vi "Graph.vi"() -> ()   [LabVIEW 2018]
panel:
  in  "Tab Control":enum32{"Page 1", "Page 2"}(tab)
  out "XY Graph":cluster{"Array Ox":dbl[], "Array Oy":dbl[]}[](graph)
  in  "Button":bool
  out "Boolean":bool
  in  "Combo Box":string(combo)
  in  "Stop":bool
  in  "Start":bool
  in  "Config":bool
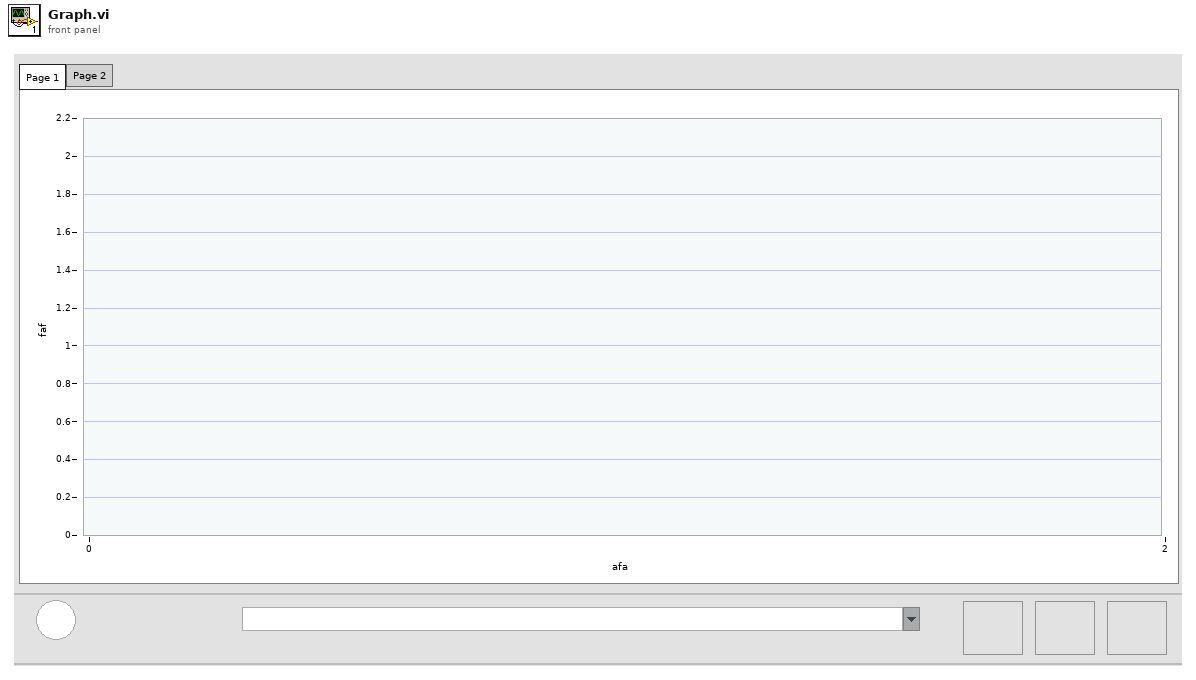
[diagram p1: front panel]
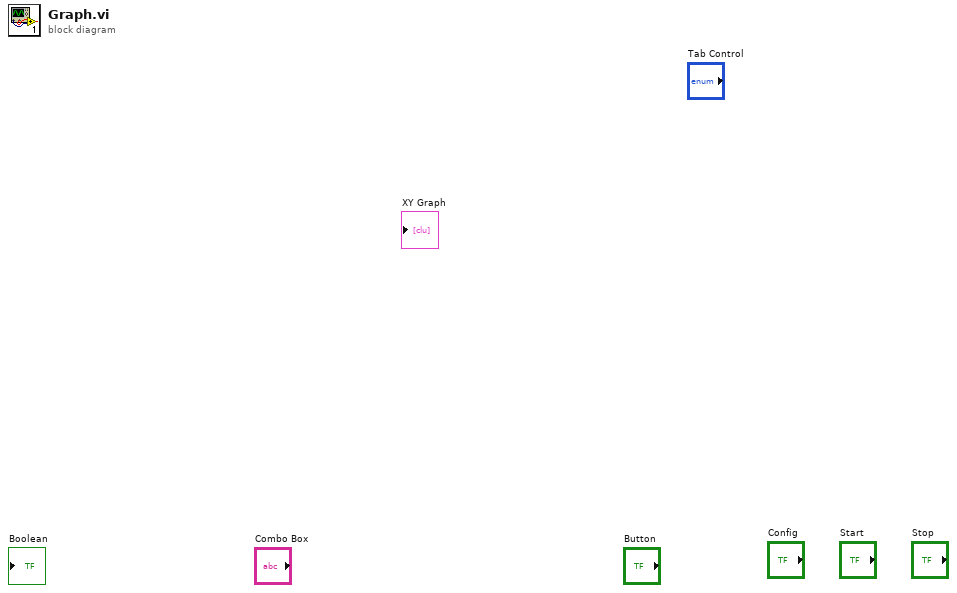
[diagram p0: block diagram]
diagram:
